vi "Write BehaviorPK.vi"(8 "error in (no error)":errorcluster, 10 "BehaviorPK":T1, 11 "BehaviorData in":refnum<class "BehaviorData.lvclass">) -> (0 "error out":errorcluster, 3 "BehaviorData out":refnum<class "BehaviorData.lvclass">)   [LabVIEW 2012, in "AcquisitionCoreLibrary.lvlib" / "BehaviorData.lvclass"]
uses:
  BehaviorData.lvclass
  Database/BehPrimary.ctl
  BehaviorData.lvclass/BehaviorData.ctl
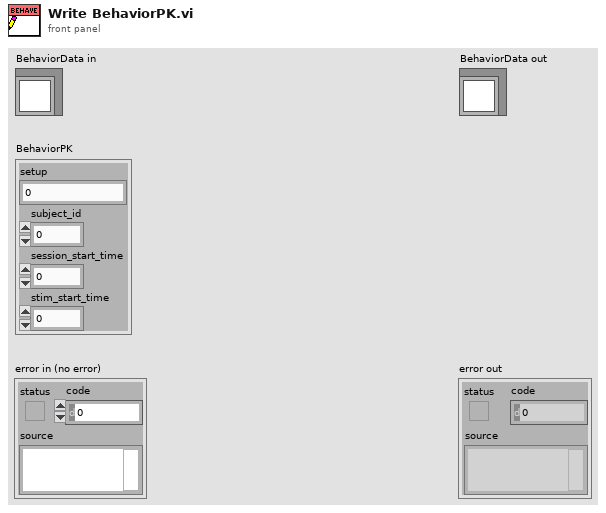
[diagram p1: front panel]
types:
  T1 = typedef "BehPrimary.ctl" = cluster{"setup":u8, "subject_id":i32, "session_start_time":dbl, "stim_start_time":dbl}
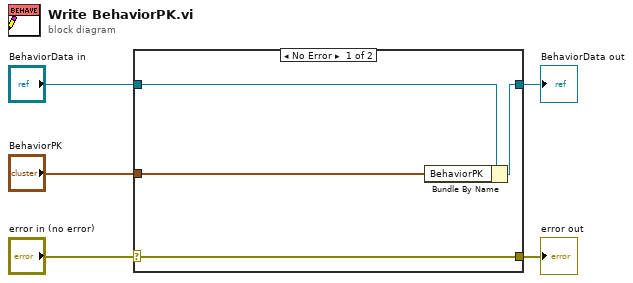
[diagram p0: block diagram]
diagram:
  n1 = case shown="No Error" "error in (no error)" {
    selector: "error in (no error)" -> [w9 w10]
    tunnel: [w9 w10] -> w4
    tunnel: [w7 w11] -> w2
    tunnel: "BehaviorData in" -> [w8 w11]
    tunnel: "BehaviorPK" -> [w6 _]
    frame No Error {
      n2 = Bundle By Name(cluster=w8, "BehaviorPK"=w6) -> (w7:refnum<class "BehaviorData.lvclass">)
    }
    frame Error {
    }
  }
  "error out" <- w4
  "BehaviorData out" <- w2
